vi "RO SM.vi"() -> ()   [LabVIEW 2013]
doc: "Use this template to build a standard state machine design pattern. Each state executes code and determines which state to transition to. Contrast this design pattern with the User Interface Event Handler pattern, in which code executes in response to user actions. Contrast this design pattern also with the Queued Message Handler pattern, in which each message handling code can queue zero or more new messages.\nNote: This template does not contain the most recent programming guidelines recommended by National Instruments. For a complete, project-based implementation of the Standard State Machine pattern, use the Create Project dialog box instead of this template."
uses:
  RO SM.ctl
panel:
  out "Beginning State":T1
  out "error out":errorcluster
  in  "error in (no error)":errorcluster
  out "Water":string
  in  "on/off":bool
  in  "Dispense":bool
  out "Indicator":cluster{"Red":bool, "Yellow":bool, "Green":bool}
  # "Red- Receive Water\nYellow-Process Water\nGreen- Ready to dispense\nwater"
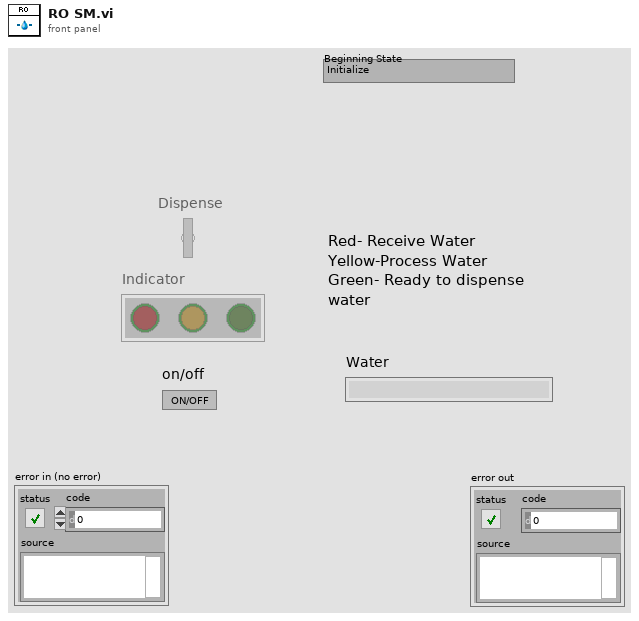
[diagram p1: front panel]
types:
  T1 = typedef "RO SM.ctl" = enum16{"Initialize", "Wait For Initialize", "Start", "Receive Water", "Process Water", "Signal Water Ready", "Wait For Dispense", "Dispense Water", "Stop"}
  T2 = enum8{"Enabled", "Disabled", "Disabled and Grayed Out"}
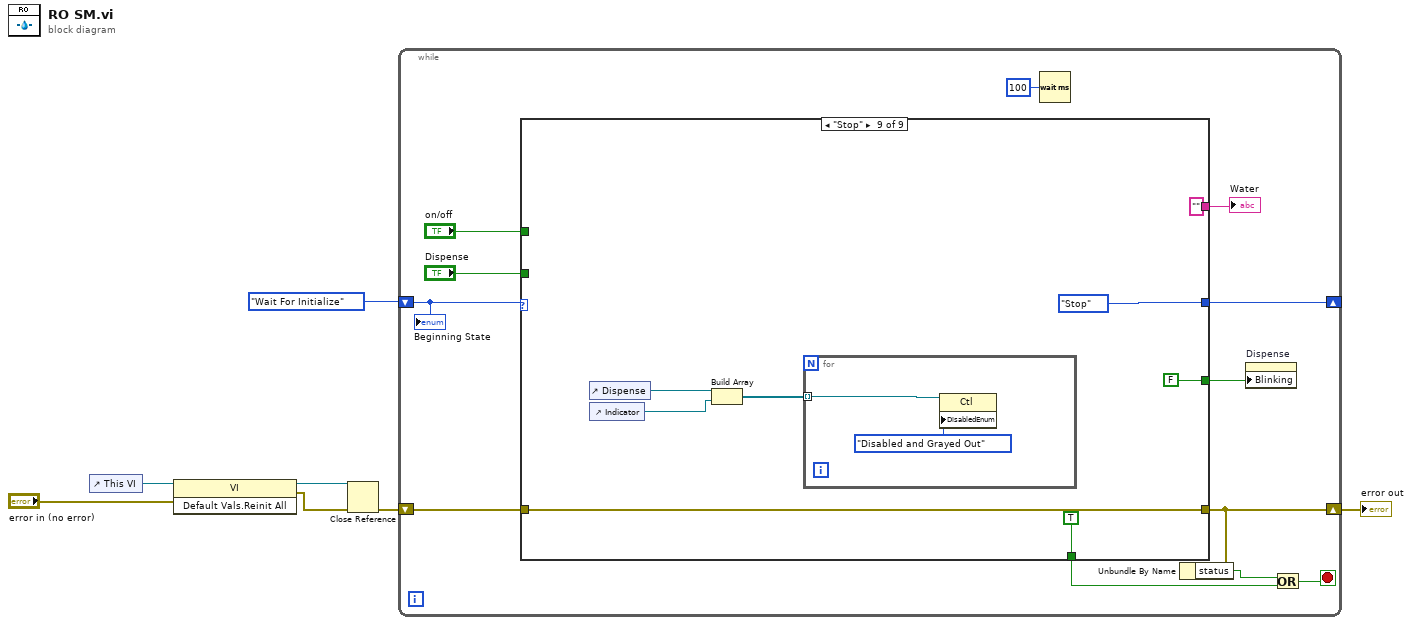
[diagram p0: block diagram]
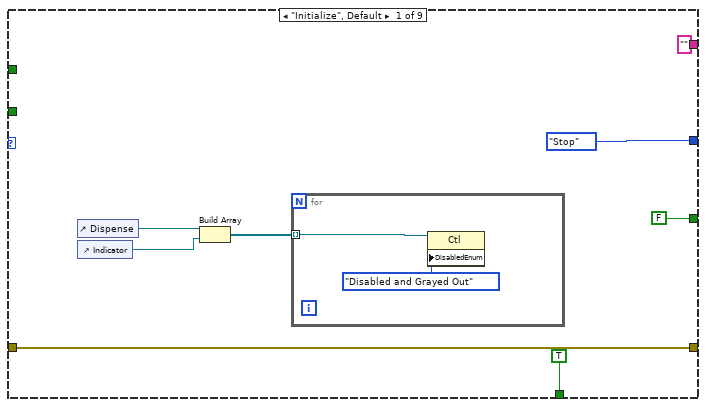
[diagram p2: hidden frame]
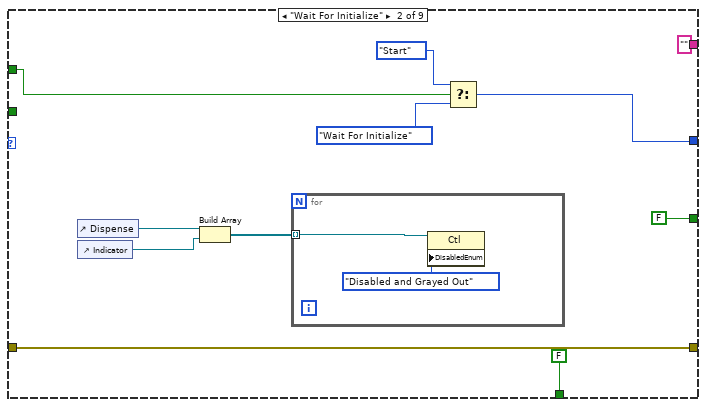
[diagram p3: hidden frame]
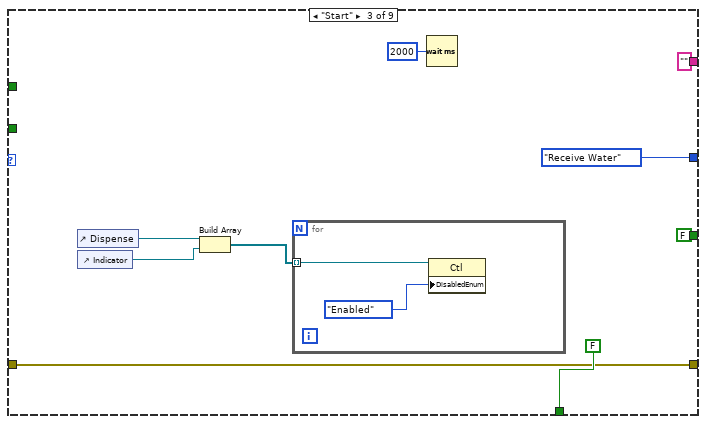
[diagram p4: hidden frame]
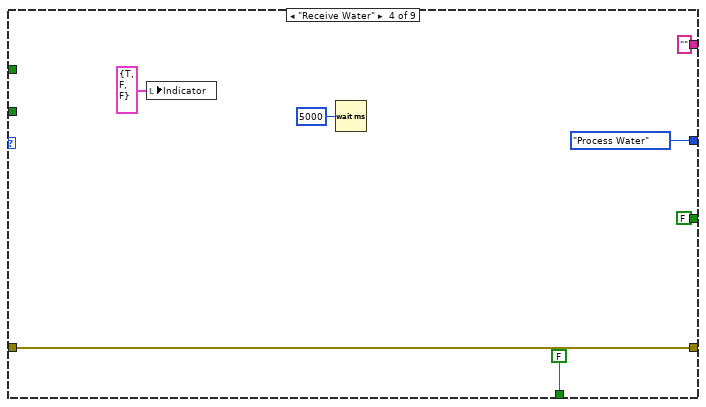
[diagram p5: hidden frame]
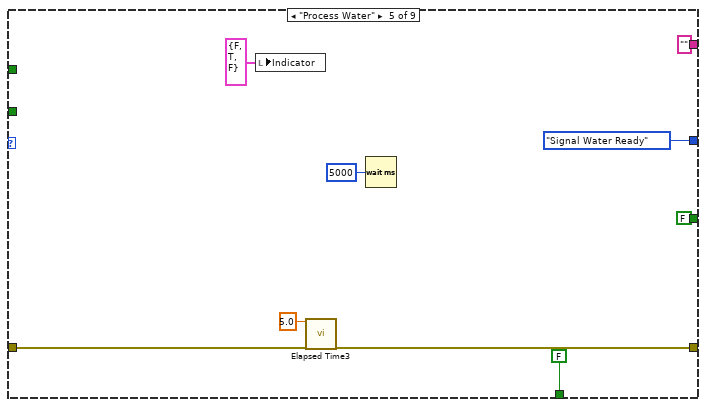
[diagram p6: hidden frame]
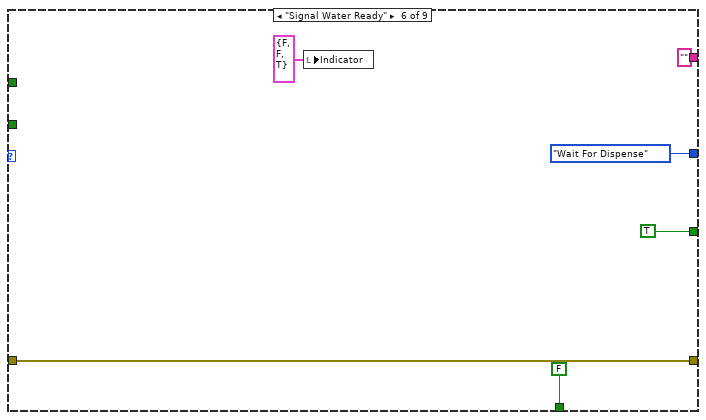
[diagram p7: hidden frame]
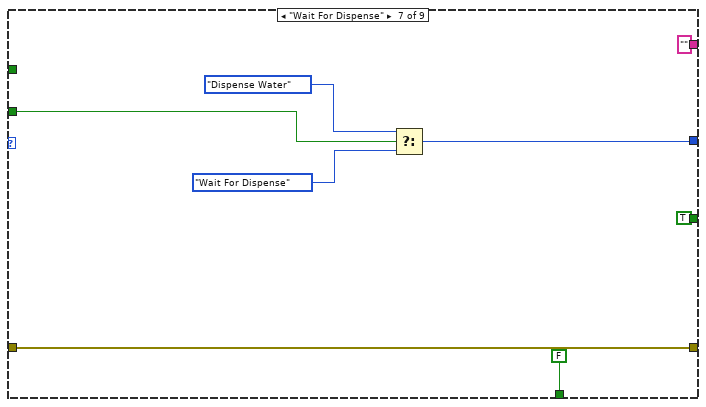
[diagram p8: hidden frame]
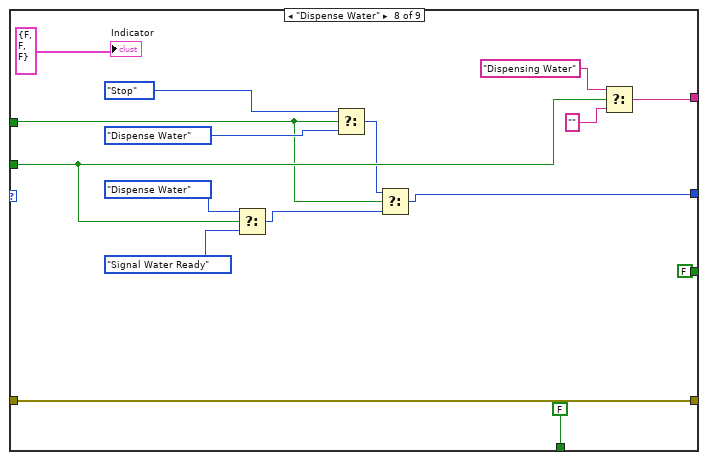
[diagram p9: hidden frame]
diagram:
  n1 = control-ref of="This VI"() -> (w6:refnum<vi>)
  n2 = invoke class="VI" method="Default Vals.Reinit All"(reference=w6, error in="error in (no error)") -> (reference out=w5:refnum<vi>, error out=w4:errorcluster)  [unwired: 1 in, 1 out]
  n3 = Close Reference(reference=w5, error in (no error)=w4) -> (error out=w2:errorcluster)
  n4 = while {
    shift-right: [w18] -> _
    shift-left: RO_SM."Wait For Initialize" ("Beginning State") -> [w19]
    shift-right: [w12] -> w1
    shift-left: w2 -> [w16]
    stop <- w10 stop-if-true
    n5 = case shown="\"Stop\"" w19 {
      tunnel: [RO_SM."Stop" ("Next State") w30 RO_SM."Receive Water" ("Next State") RO_SM."Process Water" ("Next State") RO_SM."Signal Water Ready" ("Next State") RO_SM."Wait For Dispense" ("Next State") w80 w84 RO_SM."Stop" ("Next State")] -> w18
      tunnel: [w24 w37 w43 w57 w68 w71 w79 w96 w104] -> w12
      tunnel: w16 -> [w24 w37 w43 w57 w69 w71 w79 w96 w104]
      tunnel: "on/off" -> [_ w33 _ _ _ _ _ w87 _]
      tunnel: "Dispense" -> [_ _ _ _ _ _ w83 w90 _]
      tunnel: ["" ("f") "" ("f") "" ("f") "" ("f") "" ("f") "" ("f") "" ("f") w99 "" ("f")] -> w13
      tunnel: [TRUE FALSE FALSE FALSE FALSE FALSE FALSE FALSE TRUE] -> w9
      tunnel: [FALSE FALSE FALSE FALSE FALSE TRUE TRUE FALSE FALSE] -> w8
      frame "Initialize", Default {
        n6 = control-ref of="Dispense"() -> (w27:refnum<vi>)
        n7 = control-ref of="Indicator"() -> (w26:refnum<vi>)
        n8 = Build Array(w27, w26) -> (w25:refnum<vi>[])
        n9 = for {
          tunnel: w25 -> [w29] mode=indexing
          n10 = property class="Ctl"(reference=w29, "DisabledEnum"=T2."Disabled and Grayed Out" ("Disabled")) -> ()  [unwired: 1 in, 2 out]
        }
      }
      frame "Wait For Initialize" {
        n11 = control-ref of="Dispense"() -> (w40:refnum<vi>)
        n12 = control-ref of="Indicator"() -> (w39:refnum<vi>)
        n13 = Build Array(w40, w39) -> (w38:refnum<vi>[])
        n14 = for {
          tunnel: w38 -> [w42] mode=indexing
          n15 = property class="Ctl"(reference=w42, "DisabledEnum"=T2."Disabled and Grayed Out" ("Disabled")) -> ()  [unwired: 1 in, 2 out]
        }
        n16 = Select(t=RO_SM."Start" ("Next State"), s=w33, f=RO_SM."Wait For Initialize") -> (s? t:f=w30:T1)
      }
      frame "Start" {
        n17 = control-ref of="Dispense"() -> (w50:refnum<vi>)
        n18 = control-ref of="Indicator"() -> (w49:refnum<vi>)
        n19 = Build Array(w50, w49) -> (w48:refnum<vi>[])
        n20 = for {
          tunnel: w48 -> [w53] mode=indexing
          n21 = property class="Ctl"(reference=w53, "DisabledEnum"=T2."Enabled" ("Disabled")) -> ()  [unwired: 1 in, 2 out]
        }
        n22 = Wait (ms)(milliseconds to wait=u32 2000) -> ()  [unwired: 1 out]
      }
      frame "Receive Water" {
        n23 = local write "Indicator"(cluster{"Red":bool, "Yellow":bool, "Green":bool} {"Red"=TRUE, "Yellow"=FALSE, "Green"=FALSE} ("Indicator")) -> ()
        n24 = Wait (ms)(milliseconds to wait=u32 5000) -> ()  [unwired: 1 out]
      }
      frame "Process Water" {
        n25 = local write "Indicator"(cluster{"Red":bool, "Yellow":bool, "Green":bool} {"Red"=FALSE, "Yellow"=TRUE, "Green"=FALSE} ("Indicator")) -> ()
        n26 = call "Elapsed Time3"("Time Target (s)"=5.0, "error in (no error)"=w69) -> ("error out"=w68:errorcluster)  [unwired: 10 in, 7 out]
        n27 = Wait (ms)(milliseconds to wait=u32 5000) -> ()  [unwired: 1 out]
      }
      frame "Signal Water Ready" {
        n28 = local write "Indicator"(cluster{"Red":bool, "Yellow":bool, "Green":bool} {"Red"=FALSE, "Yellow"=FALSE, "Green"=TRUE} ("Indicator")) -> ()
      }
      frame "Wait For Dispense" {
        n29 = Select(t=RO_SM."Dispense Water" ("Beginning State"), s=w83, f=RO_SM."Wait For Dispense") -> (s? t:f=w80:T1)
      }
      frame "Dispense Water" {
        n30 = Select(t=RO_SM."Dispense Water" ("Beginning State"), s=w90, f=RO_SM."Signal Water Ready" ("Beginning State")) -> (s? t:f=w85:T1)
        n31 = Select(t=RO_SM."Stop" ("Beginning State"), s=w87, f=RO_SM."Dispense Water") -> (s? t:f=w86:T1)
        n32 = Select(t=w86, s=w87, f=w85) -> (s? t:f=w84:T1)
        n33 = Select(t="Dispensing Water", s=w90, f="") -> (s? t:f=w99:string)
        "Indicator" <- cluster{"Red":bool, "Yellow":bool, "Green":bool} {"Red"=FALSE, "Yellow"=FALSE, "Green"=FALSE} ("Indicator")
      }
      frame "Stop" {
        n34 = control-ref of="Dispense"() -> (w107:refnum<vi>)
        n35 = control-ref of="Indicator"() -> (w106:refnum<vi>)
        n36 = Build Array(w107, w106) -> (w105:refnum<vi>[])
        n37 = for {
          tunnel: w105 -> [w109] mode=indexing
          n38 = property class="Ctl"(reference=w109, "DisabledEnum"=T2."Disabled and Grayed Out" ("Disabled")) -> ()  [unwired: 1 in, 2 out]
        }
      }
    }
    "Water" <- w13
    n39 = Wait (ms)(milliseconds to wait=u32 100) -> ()  [unwired: 1 out]
    n40 = Unbundle By Name(w12) -> ("status"=w11:bool)
    n41 = property on="Dispense" class="Bool (strict)"("Blinking"=w8) -> ()  [unwired: 2 in, 2 out]
    n42 = Or(x=w11, y=w9) -> (x .or. y?=w10:bool)
    "Beginning State" <- w19
  }
  "error out" <- w1
